vi "Search & Replace Sub-String.vi"() -> ()   [LabVIEW 2016]
panel:
  out "error out":errorcluster
  out "offset past replacement":i32
  out "number of replacements":i32
  out "result string":string
  in  "error in (no error)":errorcluster
  in  "offset (0)":i32
  in  "replace string (\"\")":string
  in  "search string":string
  in  "ignore case? (F)":bool
  in  "replace all? (F)":bool
  in  "input string":string
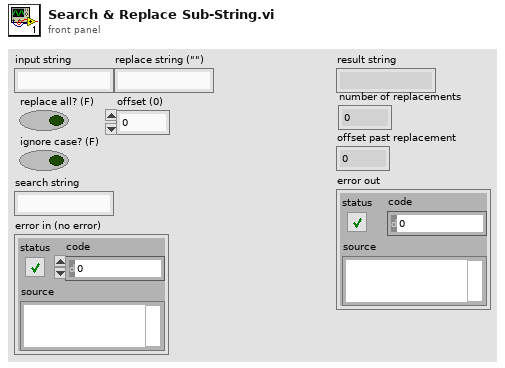
[diagram p1: front panel]
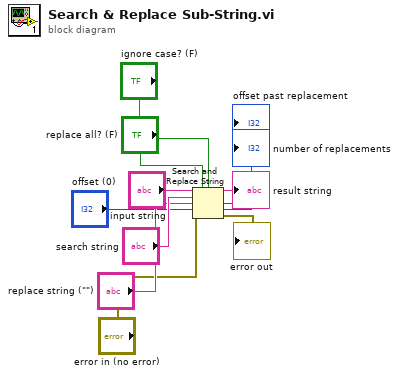
[diagram p0: block diagram]
diagram:
  n1 = Search and Replace String(replace all?="replace all? (F)", case sensitive?="ignore case? (F)", input string="input string", search string="search string", replace string="replace string (\"\")", offset="offset (0)", error in="error in (no error)") -> (result string=→"result string":string, number of replacements=→"number of replacements":i32, offset past replacement=→"offset past replacement":i32, error out=→"error out":errorcluster)  [unwired: 1 in]
